vi "Update Channel Benchmark.vi"(7 "Reinit":bool, 8 "error in (no error)":errorcluster, 9 "X0":i64, 10 "X1":i64, 11 "CIFChannels in":refnum<class "CIFChannels.lvclass">) -> (0 "error out":errorcluster, 3 "CIFChannels out":refnum<class "CIFChannels.lvclass">)   [LabVIEW 2021, in "CIFChannels.lvclass"]
doc: "Load a new data value into the statistics class for the channel. The new value will be calculated by subracting the X0 value from the X1 value. This VI is intended to benchmark the amount of time spent reading/writing the channel values."
uses:
  CIFChannels.lvclass
  CIFChannels.lvclass/CIFChannels.ctl
  <vilib>/CIF Foundation/CIF Utilities/Statistics/I64/Stats_I64_CIF_U.lvclass
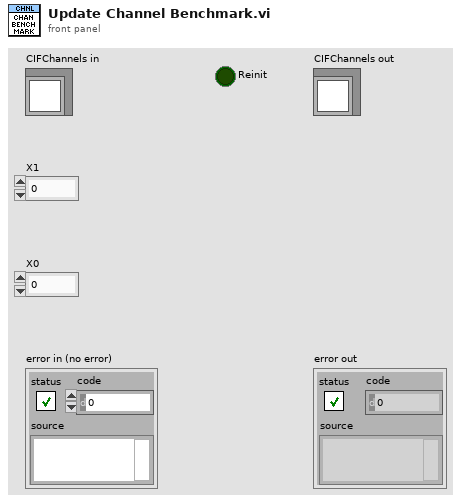
[diagram p1: front panel]
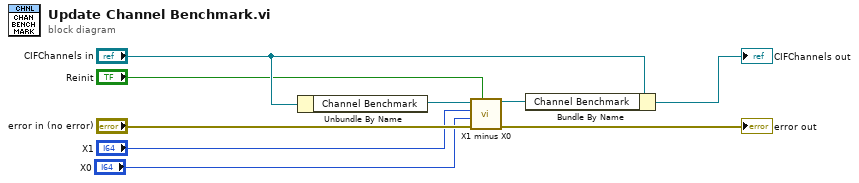
[diagram p0: block diagram]
diagram:
  n1 = Unbundle By Name("CIFChannels in") -> ("Channel Benchmark"=w5:refnum<class "Stats_I64_CIF_U.lvclass">)
  n2 = call <vilib>:"X1 minus X0.vi"("Reinit"="Reinit", "error in (no error)"="error in (no error)", "X0"="X0", "X1"="X1", "Stats_I64_CIF_U in"=w5) -> ("error out"=→"error out":errorcluster, "Stats_I64_CIF_U out"=w4:refnum<class "Stats_I64_CIF_U.lvclass">)  [unwired: 5 in]
  n3 = Bundle By Name(cluster="CIFChannels in", "Channel Benchmark"=w4) -> (→"CIFChannels out":refnum<class "CIFChannels.lvclass">)
